vi "1_SimpleDemo_TH260Histo.vi"() -> ()   [LabVIEW 2010]
uses:
  _lib/PQ/TimeHarp260/th260lib_x86_x64_UIThread.llb/TH260_DllPath_global.vi
  _lib/PQ/TimeHarp260/TH260_LibVersion_global.vi
  _lib/PQ/TimeHarp260/TH260_MeasMode.ctl
  _lib/PQ/TimeHarp260/TH260_TimingMode.ctl
panel:
  in  "dtcode":i32(ring) caption="Deadtime  [ns]" items=["24", "44", "66", "88", "112", "135", "160", "180"]
  in  "TrgLevel":i32=-100 caption="Trg.Level [mV]" min=-1200 max=1200 step=1
  in  "TrgEdge":i32(ring) items=["falling", "rising"]
  in  "SyncTrgEdge":i32(ring) caption="TrgEdge" items=["falling", "rising"]
  in  "SyncTrgLevel":i32=-100 caption="Trg.Level [mV]" min=-1200 max=1200 step=1
  in  "Binning":i32(ring) caption="Resolution [ps]" items=["25.000000", "50.000000", "100.000000", "200.000000", "400.000000", "800.000000", "1600.000000", "3200.000000", "6400.000000", "12800.000000", "25600.000000", "51200.000000", "102400.000000", "204800.000000", "409600.000000", "819200.000000", "1638400.000000", "3276800.000000", "6553600.000000", "13107200.000000", "26214400.000000", "52428800.000000"]
  in  "HistoLength":i32(ring)=5 caption="Histo Length" items=["1024", "2048", "4096", "8192", "16384", "32768"]
  in  "Acqu.Time":i32=10000 caption="Acqu.Time [ms]" min=1 max=360000000 step=1
  in  "GlobalOffset":i32 caption="GlobalOffset [ns]" min=0 max=100000000 step=1
  in  "OverflowLevel":u32=65535 min=1 step=1
  in  "StopOnOverflow":bool=TRUE
  in  "InputZeroX":i32=-10 caption="ZeroCr. [mV]" min=-40 max=0 step=1
  in  "InputCFDLevel":i32=-100 caption="CFDLevel [mV]" min=-1200 max=0 step=1
  in  "Offset":i32 caption="Offset [ps]" min=-99999 max=99999 step=1
  in  "Enable":bool=TRUE
  in  "SyncZeroX":i32=-10 caption="ZeroCr. [mV]" min=-40 max=0 step=1
  in  "SyncCFDLevel":i32=-100 caption="CFDLevel [mV]" min=-1200 max=0 step=1
  in  "SyncOffset":i32 caption="SyncOffset [ps]" min=-99999 max=99999 step=1
  in  "SyncDivider":i32(ring)=8 items=["1"=1, "2"=2, "4"=4, "8"=8]
  out "HistoGraph":T1(graph)={0.0, "Resolution"=0.025, "Histogram"=array2x32768[65536 elements]}
  out "CountRates":i32[](array[numeric]) caption="Count Rates [cps]"
  out "SyncRate":i32 caption="Sync Rate [cps]"
  in  "stop":bool
  out "error out":errorcluster
  # "Acquisition"
  # "All Channels"
  # "Sync"
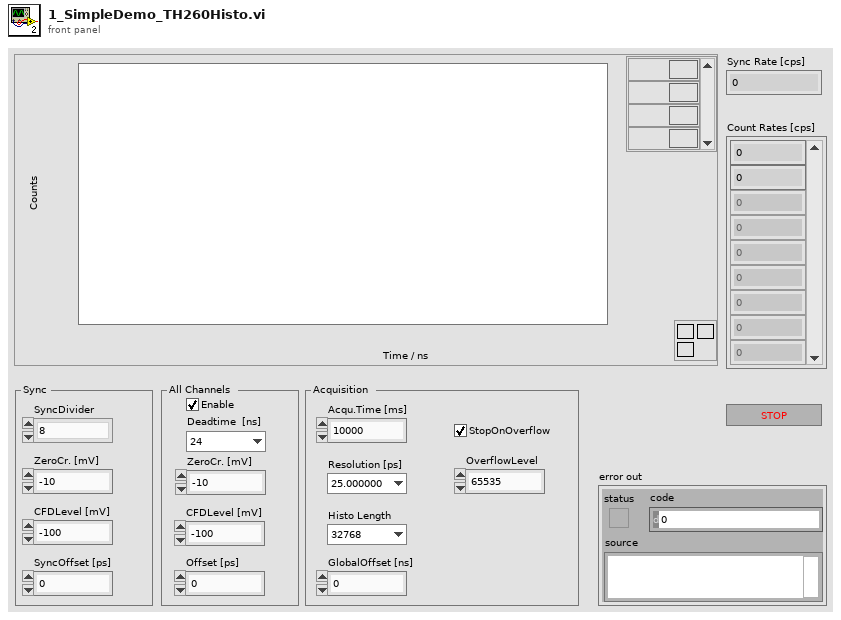
[diagram p1: front panel]
types:
  T1 = cluster{dbl, "Resolution":dbl, "Histogram":u32[][]}
  T2 = typedef "TH260_TimingMode.ctl" = i32
  T3 = typedef "TH260_MeasMode.ctl" = i32
  T4 = typedef "TH260_InitInfo.ctl" = cluster{"Library Version":string, "Serial No.":string, "Model":string, "Partnum":string, "Version":string, "features":i32, "nchannels":i32, "Base Resolution":dbl, "Bin Steps":i32}
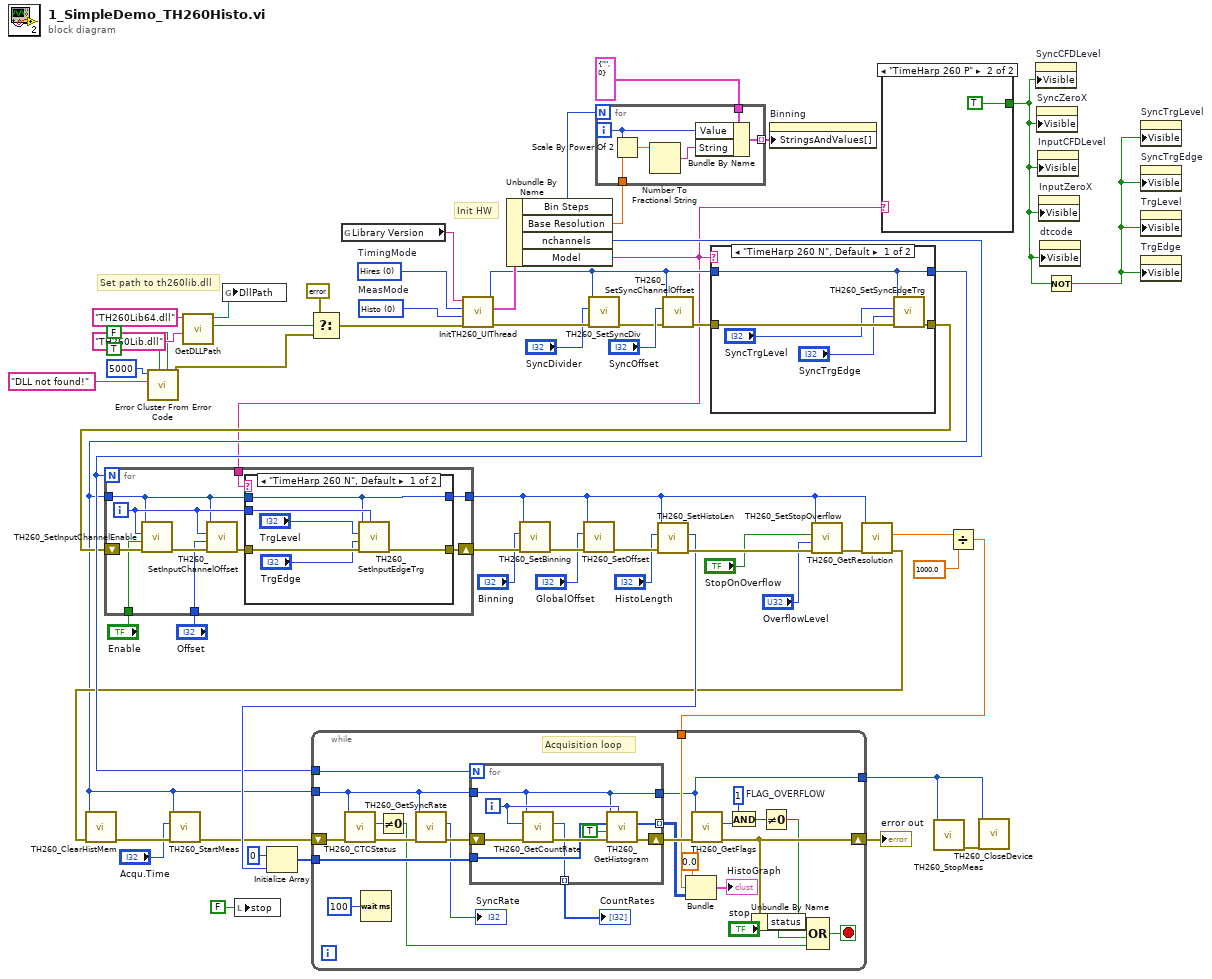
[diagram p0: block diagram]
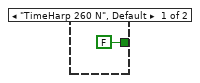
[diagram p2: hidden frame]
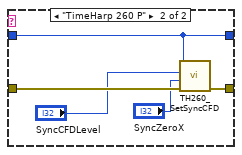
[diagram p3: hidden frame]
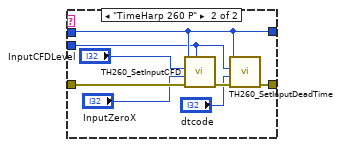
[diagram p4: hidden frame]
diagram:
  w8 = T2 0 items=["Hires", "Lowres"]  # TimingMode
  w58 = T3 0 items=["Histo"=0, "T2"=2, "T3"=3]  # MeasMode
  # "Init HW"
  # "Set path to th260lib.dll"
  n1 = call <vilib>:"Error Cluster From Error Code.vi"("is warning? (False)"=FALSE, "show call chain? (False)"=TRUE, "error message (\"\")"="DLL not found!" ("error message (\"\")"), "error code (0)"=5000) -> ("error out"=w57:errorcluster)  [unwired: 5 in]
  n2 = call "GetDLLPath.vi"("DllName_32bit"="TH260Lib.dll" ("name or relative path"), "DllName_64bit"="TH260Lib64.dll" ("name or relative path")) -> ("file exists?"=w55:bool, "DLLPath"=w54:path)  [unwired: 8 in]
  n3 = global write "TH260_DllPath_global.vi" "DllPath"(w54) -> ()
  n4 = local write "stop"(FALSE ("stop")) -> ()
  n5 = Select(t=errorcluster {"status"=FALSE, "code"=0, "source"=""} ("error IO"), s=w55, f=w57) -> (s? t:f=w51:errorcluster)
  n6 = global read "TH260_LibVersion_global.vi" "Library Version"() -> (w16:string)
  n7 = call "InitTH260_UIThread.vi"("error in (no error)"=w51, "MeasMode"=w58, "TimingMode"=w8, "Library Version"=w16) -> ("error out"=w46:errorcluster, "Init Info"=w48:T4, "DevIdx"=w20:i32)  [unwired: 5 in]
  n8 = Unbundle By Name(w48) -> ("Bin Steps"=w12:i32, "Base Resolution"=w9:dbl, "nchannels"=w28:i32, "Model"=w7:string)
  n9 = call "TH260_SetSyncDiv.vi"("error in (no error)"=w46, "SyncDivider"="SyncDivider", "devidx"=w20) -> ("error out"=w45:errorcluster)  [unwired: 7 in, 1 out]
  n10 = for {
    N: w12 -> [_]
    tunnel: cluster{"String":string, "Value":i32} {"String"="", "Value"=0} -> [w64]
    tunnel: [w63] -> w10 mode=indexing
    tunnel: w9 -> [w62]
    i -> [w61]
    n11 = Scale By Power Of 2(n=w61, x=w62) -> (x*2^n=w60:dbl)
    n12 = Number To Fractional String(number=w60) -> (F-format string=w59:string)  [unwired: 3 in]
    n13 = Bundle By Name(cluster=w64, "Value"=w61, "String"=w59) -> (w63:cluster{"String":string, "Value":i32})
  }
  n14 = call "TH260_SetSyncChannelOffset.vi"("error in (no error)"=w45, "Offset"="SyncOffset", "devidx"=w20) -> ("error out"=w49:errorcluster)  [unwired: 7 in, 1 out]
  n15 = case shown="\"TimeHarp 260 N\", Default" w7 {
    tunnel: w49 -> [w69 w74]
    tunnel: [w68 w72] -> w27
    tunnel: w20 -> [w67 w70]
    tunnel: [w67 w70] -> w13
    frame "TimeHarp 260 N", Default {
      n16 = call "TH260_SetSyncEdgeTrg.vi"("error in (no error)"=w69, "edge"="SyncTrgEdge", "level"="SyncTrgLevel", "devidx"=w67) -> ("error out"=w68:errorcluster)  [unwired: 6 in, 1 out]
    }
    frame "TimeHarp 260 P" {
      n17 = call "TH260_SetSyncCFD.vi"("error in (no error)"=w74, "CFD ZeroCross"="SyncZeroX", "CFD Level"="SyncCFDLevel", "devidx"=w70) -> ("error out"=w72:errorcluster)  [unwired: 6 in, 1 out]
    }
  }
  n18 = for {
    N: w28 -> [_]
    shift-right: [w81] -> w47
    shift-left: w27 -> [w84]
    tunnel: w13 -> [w79]
    tunnel: [w76] -> w23
    tunnel: "Enable" -> [w78]
    tunnel: "Offset" -> [w77]
    tunnel: w7 -> [w75]
    i -> [w80]
    n19 = call "TH260_SetInputChannelEnable.vi"("error in (no error)"=w84, "enable"=w78, "channel"=w80, "devidx"=w79) -> ("error out"=w83:errorcluster)  [unwired: 6 in, 1 out]
    n20 = call "TH260_SetInputChannelOffset.vi"("error in (no error)"=w83, "offset"=w77, "channel"=w80, "devidx"=w79) -> ("error out"=w82:errorcluster)  [unwired: 6 in, 1 out]
    n21 = case shown="\"TimeHarp 260 N\", Default" w75 {
      tunnel: w82 -> [w90 w98]
      tunnel: [w89 w94] -> w81
      tunnel: w80 -> [w88 w92]
      tunnel: w79 -> [w87 w93]
      tunnel: [w87 w93] -> w76
      frame "TimeHarp 260 N", Default {
        n22 = call "TH260_SetInputEdgeTrg.vi"("channel"=w88, "error in (no error)"=w90, "edge"="TrgEdge", "level"="TrgLevel", "devidx"=w87) -> ("error out"=w89:errorcluster)  [unwired: 5 in, 1 out]
      }
      frame "TimeHarp 260 P" {
        n23 = call "TH260_SetInputCFD.vi"("channel"=w92, "error in (no error)"=w98, "CFD ZeroCross"="InputZeroX", "CFD Level"="InputCFDLevel", "devidx"=w93) -> ("error out"=w95:errorcluster)  [unwired: 5 in, 1 out]
        n24 = call "TH260_SetInputDeadTime.vi"("error in (no error)"=w95, "dtcode"="dtcode", "channel"=w92, "devidx"=w93) -> ("error out"=w94:errorcluster)  [unwired: 6 in, 1 out]
      }
    }
  }
  n25 = call "TH260_SetBinning.vi"("error in (no error)"=w47, "Binning"="Binning", "devidx"=w23) -> ("error out"=w43:errorcluster)  [unwired: 7 in, 1 out]
  n26 = call "TH260_SetOffset.vi"("error in (no error)"=w43, "Offset"="GlobalOffset", "devidx"=w23) -> ("error out"=w41:errorcluster)  [unwired: 7 in, 1 out]
  n27 = call "TH260_SetHistoLen.vi"("error in (no error)"=w41, "lencode"="HistoLength", "devidx"=w23) -> ("error out"=w40:errorcluster, "actuallen"=w33:i32)  [unwired: 6 in, 1 out]
  n28 = Initialize Array(u32 0, w33) -> (w32:u32[])
  n29 = property on="Binning" class="Ring (strict)"("StringsAndValues[]"=w10) -> ()  [unwired: 2 in, 2 out]
  n30 = call "TH260_SetStopOverflow.vi"("error in (no error)"=w40, "stopcount"="OverflowLevel", "StopOnOverflow"="StopOnOverflow", "devidx"=w23) -> ("error out"=w24:errorcluster)  [unwired: 6 in, 1 out]
  n31 = call "TH260_GetResolution.vi"("error in (no error)"=w24, "devidx"=w23) -> ("error out"=w21:errorcluster, "resolution"=w22:dbl)  [unwired: 7 in, 1 out]
  n32 = call "TH260_ClearHistMem.vi"("error in (no error)"=w21, "devidx"=w13) -> ("error out"=w37:errorcluster)  [unwired: 8 in, 1 out]
  n33 = call "TH260_StartMeas.vi"("error in (no error)"=w37, "Acquisition time"="Acqu.Time", "devidx"=w13) -> ("error out"=w19:errorcluster)  [unwired: 7 in, 1 out]
  n34 = case shown="\"TimeHarp 260 P\"" w7 {
    tunnel: [FALSE ("Visible") TRUE ("Visible")] -> w6
    frame "TimeHarp 260 N", Default {
    }
    frame "TimeHarp 260 P" {
    }
  }
  n35 = Divide(x=w22, y=1000.0) -> (x/y=w29:dbl)
  n36 = while {
    shift-right: [w113] -> w35
    shift-left: w19 -> [w124]
    tunnel: w13 -> [w120]
    tunnel: w28 -> [w123]
    tunnel: w32 -> [w115]
    tunnel: w29 -> [w107]
    tunnel: [w102] -> w15
    stop <- w114 stop-if-true
    w118 = 1  # FLAG_OVERFLOW
    # "Acquisition loop"
    n37 = call "TH260_CTCStatus.vi"("error in (no error)"=w124, "devidx"=w120) -> ("error out"=w122:errorcluster, "ctcstatus"=w125:i32)  [unwired: 7 in, 1 out]
    n38 = Wait (ms)(milliseconds to wait=u32 100) -> ()  [unwired: 1 out]
    n39 = Not Equal To 0?(x=w125) -> (x != 0?=w104:bool)
    n40 = call "TH260_GetSyncRate.vi"("error in (no error)"=w122, "devidx"=w120) -> ("error out"=w121:errorcluster, "rate"=→"SyncRate":i32)  [unwired: 7 in, 1 out]
    n41 = for {
      N: w123 -> [_]
      shift-right: [w134] -> w119
      shift-left: w121 -> [w133]
      tunnel: w120 -> [w130]
      tunnel: [w130] -> w102
      tunnel: w115 -> [w129]
      tunnel: [w128] -> w110 mode=indexing
      tunnel: [w127] -> w109 mode=indexing
      i -> [w131]
      n42 = call "TH260_GetCountRate.vi"("error in (no error)"=w133, "Channel"=w131, "devidx"=w130) -> ("error out"=w132:errorcluster, "rate"=w128:i32)  [unwired: 6 in, 1 out]
      n43 = call "TH260_GetHistogram.vi"("devidx"=w130, "Buffer"=w129, "clear"=TRUE, "error in (no error)"=w132, "channel"=w131) -> ("Histogram"=w127:u32[], "error out"=w134:errorcluster)  [unwired: 3 in, 1 out]
    }
    "CountRates" <- w110
    n44 = Bundle(0.0, w107, "Histogram"=w109) -> (→"HistoGraph":cluster{dbl, dbl, "Histogram":u32[][]})  [unwired: 1 in]
    n45 = call "TH260_GetFlags.vi"("error in (no error)"=w119, "devidx"=w102) -> ("error out"=w113:errorcluster, "flags"=w116:i32)  [unwired: 7 in, 1 out]
    n46 = And(x=w118, y=w116) -> (x .and. y?=w117:i32)
    n47 = Unbundle By Name(w113) -> ("status"=w101:bool)
    n48 = Not Equal To 0?(x=w117) -> (x != 0?=w112:bool)
    n49 = Compound Arithmetic op=OR(w101, w112, "stop", w104) -> (w114:bool)
  }
  "error out" <- w35
  n50 = call "TH260_StopMeas.vi"("devidx"=w15) -> ("error out"=w14:errorcluster)  [unwired: 9 in, 1 out]
  n51 = call "TH260_CloseDevice.vi"("error in (no error)"=w14, "devidx"=w15) -> ()  [unwired: 8 in, 2 out]
  n52 = property on="SyncCFDLevel" class="DigNum (strict)"("Visible"=w6) -> ()  [unwired: 2 in, 2 out]
  n53 = property on="SyncZeroX" class="DigNum (strict)"("Visible"=w6) -> ()  [unwired: 2 in, 2 out]
  n54 = property on="InputCFDLevel" class="DigNum (strict)"("Visible"=w6) -> ()  [unwired: 2 in, 2 out]
  n55 = property on="InputZeroX" class="DigNum (strict)"("Visible"=w6) -> ()  [unwired: 2 in, 2 out]
  n56 = property on="dtcode" class="Ring (strict)"("Visible"=w6) -> ()  [unwired: 2 in, 2 out]
  n57 = Not(x=w6) -> (.not. x?=w5:bool)
  n58 = property on="SyncTrgLevel" class="DigNum (strict)"("Visible"=w5) -> ()  [unwired: 2 in, 2 out]
  n59 = property on="SyncTrgEdge" class="Ring (strict)"("Visible"=w5) -> ()  [unwired: 2 in, 2 out]
  n60 = property on="TrgLevel" class="DigNum (strict)"("Visible"=w5) -> ()  [unwired: 2 in, 2 out]
  n61 = property on="TrgEdge" class="Ring (strict)"("Visible"=w5) -> ()  [unwired: 2 in, 2 out]
